vi "Cursor Values.vi"(7 "Plot":T2 items=["FRF", "rad phase unwrapped", "deg phase unwrapped", "rad phase wrapped", "deg phase wrapped", "White Plots", "MJ Map", "Real and Imaginary"], 8 "option?":bool, 9 "Start Coord":T1, 10 "Coords":T1, 11 "WaveformGraph in":refnum<vi>) -> (3 "Position":string)   [LabVIEW 2022 SP3]
uses:
  <vilib>/Utility/miscctls.llb/LVPoint32TypeDef.ctl
  GraphType.ctl
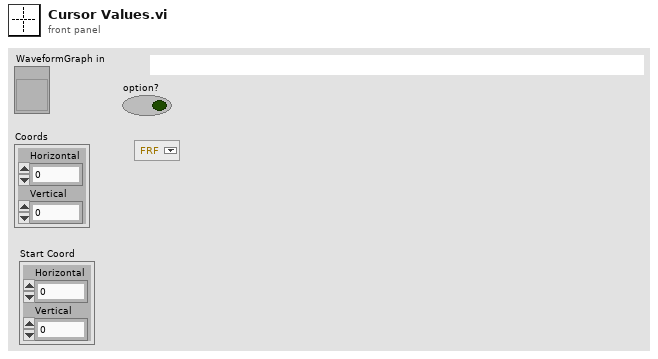
[diagram p1: front panel]
types:
  T1 = typedef "LVPoint32TypeDef.ctl" = cluster{"Horizontal":i32, "Vertical":i32}
  T2 = typedef "GraphType.ctl" = u16
  T3 = typedef "LVPointDoubleTypeDef.ctl" = cluster{"X":dbl, "Y":dbl}
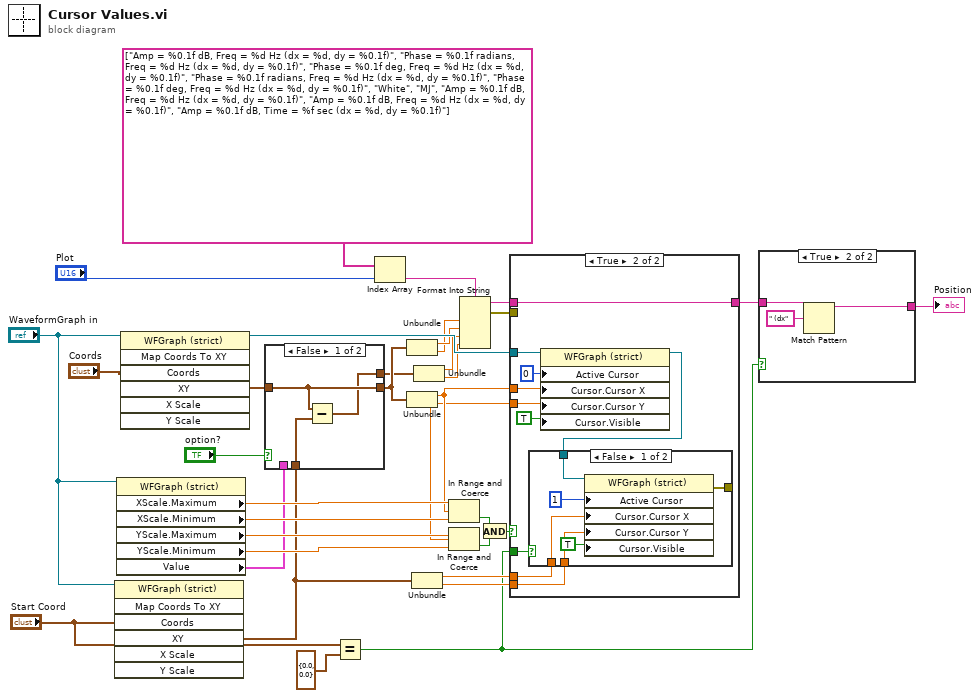
[diagram p0: block diagram]
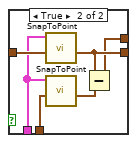
[diagram p3: hidden frame]
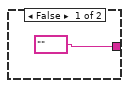
[diagram p4: hidden frame]
diagram:
  n1 = invoke class="WFGraph (strict)" method="Map Coords To XY"(reference="WaveformGraph in", "Coords"="Start Coord") -> ("XY"=w6:cluster{"X":dbl, "Y":dbl})  [unwired: 5 in, 6 out]
  n2 = property class="WFGraph (strict)"(reference="WaveformGraph in") -> ("XScale.Maximum"=w30:dbl, "XScale.Minimum"=w29:dbl, "YScale.Maximum"=w27:dbl, "YScale.Minimum"=w26:dbl, "Value"=w21:cluster{dbl, "df":dbl, dbl[]}[])  [unwired: 1 in, 2 out]
  n3 = invoke class="WFGraph (strict)" method="Map Coords To XY"(reference="WaveformGraph in", "Coords"="Coords") -> (reference out=w34:refnum<vi>, "XY"=w18:cluster{"X":dbl, "Y":dbl})  [unwired: 5 in, 5 out]
  n4 = case shown="False" "option?" {
    tunnel: w21 -> [_ w42]
    tunnel: [w37 w39] -> w13
    tunnel: w18 -> [w37 w43]
    tunnel: w6 -> [w36 w41]
    tunnel: [w35 w38] -> w12
    frame False {
      n5 = Subtract(x=w37, y=w36) -> (x-y=w35:cluster{"X":dbl, "Y":dbl})
    }
    frame True {
      n6 = call "SnapToPoint.vi"("Cursor.Cursor Position in"=w43, "Value"=w42) -> ("Cursor.Cursor Position out"=w39:T3)  [unwired: 9 in]
      n7 = call "SnapToPoint.vi"("Cursor.Cursor Position in"=w41, "Value"=w42) -> ("Cursor.Cursor Position out"=w40:T3)  [unwired: 9 in]
      n8 = Subtract(x=w39, y=w40) -> (x-y=w38:T3)
    }
  }
  n9 = Equal?(x="Start Coord", y=cluster{"X":dbl, "Y":dbl} {"X"=0.0, "Y"=0.0}) -> (x = y?=w3:bool)
  n10 = Index Array(array=string[] ["Amp = %0.1f dB, Freq = %d Hz (dx = %d, dy = %0.1f)", "Phase = %0.1f radians, Freq = %d Hz (dx = %d, dy = %0.1f)", "Phase = %0.1f deg, Freq = %d Hz (dx = %d, dy = %0.1f)", "Phase = %0.1f radians, Freq = %d Hz (dx = %d, dy = %0.1f)", "Phase = %0.1f deg, Freq = %d Hz (dx = %d, dy = %0.1f)", "White", "MJ", "Amp = %0.1f dB, Freq = %d Hz (dx = %d, dy = %0.1f)", "Amp = %0.1f dB, Freq = %d Hz (dx = %d, dy = %0.1f)", "Amp = %0.1f dB, Time = %f sec (dx = %d, dy = %0.1f)"], index="Plot") -> (element=w15:string)
  n11 = Unbundle(w13) -> ("X"=w33:dbl, "Y"=w32:dbl)
  n12 = Unbundle(w13) -> ("X"=w28:dbl, "Y"=w25:dbl)
  n13 = Unbundle(w6) -> ("X"=w5:dbl, "Y"=w4:dbl)
  n14 = Unbundle(w12) -> ("X"=w11:dbl, "Y"=w10:dbl)
  n15 = In Range and Coerce(upper limit=w30, x=w28, lower limit=w29) -> (In Range?=w23:bool)  [unwired: 1 out]
  n16 = In Range and Coerce(upper limit=w27, x=w25, lower limit=w26) -> (In Range?=w24:bool)  [unwired: 1 out]
  n17 = Format Into String(format string=w15, w32, w33, w11, w10) -> (resulting string=w31:string, error out=w1:errorcluster)  [unwired: 2 in]
  n18 = And(x=w23, y=w24) -> (x .and. y?=w22:bool)
  n19 = case shown="True" w22 {
    tunnel: w34 -> [_ w54]
    tunnel: w25 -> [_ w53]
    tunnel: w31 -> [_ w51]
    tunnel: w28 -> [_ w52]
    tunnel: ["" w51] -> w9
    tunnel: w5 -> [_ w48]
    tunnel: w4 -> [_ w47]
    tunnel: w3 -> [_ w46]
    tunnel: w1 -> [_ _]
    frame False {
    }
    frame True {
      n20 = property on="Property Node" class="WFGraph (strict)"(reference=w54, "Active Cursor"=u32 0, "Cursor.Cursor X"=w52, "Cursor.Cursor Y"=w53, "Cursor.Visible"=TRUE) -> (reference out=w49:refnum<vi>)  [unwired: 1 in, 1 out]
      n21 = case shown="False" w46 {
        tunnel: w49 -> [w59 _]
        tunnel: w48 -> [w58 _]
        tunnel: w47 -> [w57 _]
        tunnel: [w56 _] -> _
        frame False {
          n22 = property on="Property Node" class="WFGraph (strict)"(reference=w59, "Active Cursor"=u32 1, "Cursor.Cursor X"=w58, "Cursor.Cursor Y"=w57, "Cursor.Visible"=TRUE) -> (error out=w56:errorcluster)  [unwired: 1 in, 1 out]
        }
        frame True {
        }
      }
    }
  }
  n23 = case shown="True" w3 {
    tunnel: w9 -> [w61 w64]
    tunnel: [w61 w62] -> w8
    frame False {
    }
    frame True {
      n24 = Match Pattern(string=w64, regular expression=" (dx") -> (before substring=w62:string)  [unwired: 1 in, 3 out]
    }
  }
  "Position" <- w8
